vi "FormatLog.vi"(6 "log input":string, 8 "error in (no error)":errorcluster, 9 "System":string, 10 "Type":T1(ring), 11 "Log in":refnum<class "Log.lvclass">) -> (0 "error out":errorcluster, 3 "Log out":refnum<class "Log.lvclass">)   [LabVIEW 2018, in "Log.lvclass"]
uses:
  Log.lvclass
  Log.lvclass/Log.ctl
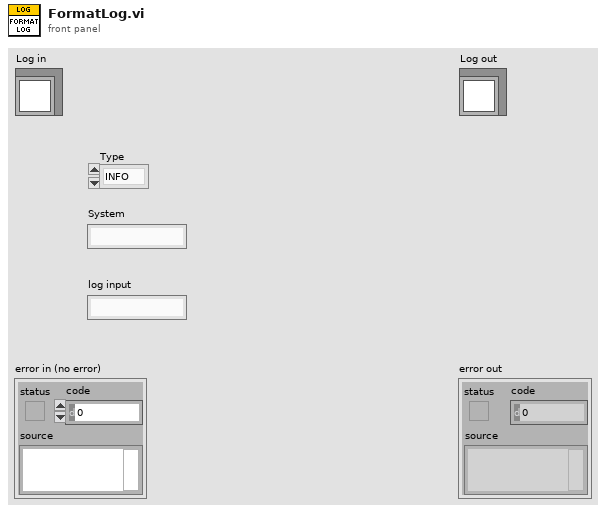
[diagram p1: front panel]
types:
  T1 = enum16{"INFO ", "TRACE", "DEBUG", "WARN ", "ERROR", "FATAL", "OTHER"}
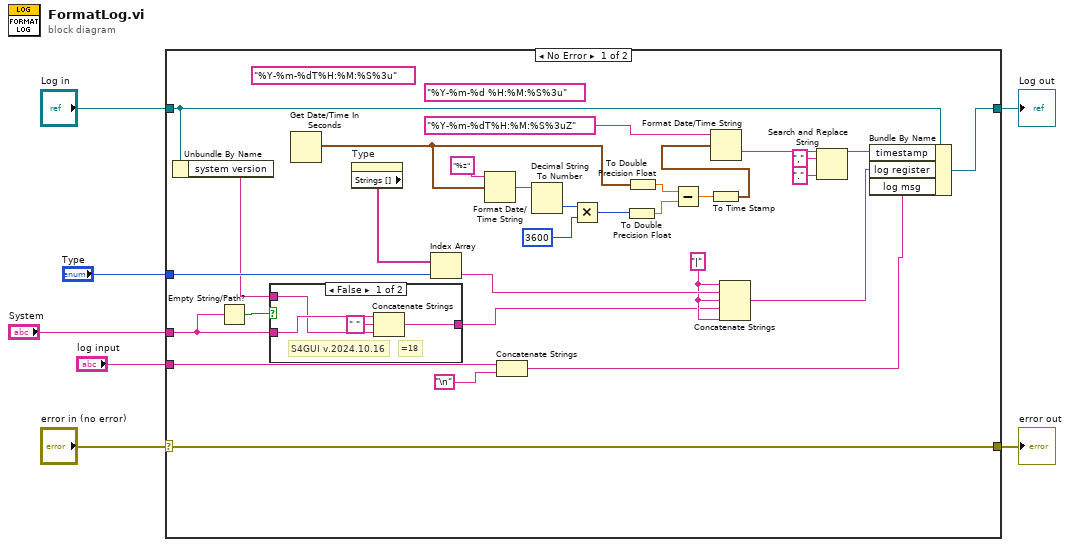
[diagram p0: block diagram]
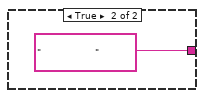
[diagram p2: hidden frame]
diagram:
  n1 = case shown="No Error" "error in (no error)" {
    selector: "error in (no error)" -> [w37 w44]
    tunnel: [w37 w44] -> w6
    tunnel: [w31 w43] -> w5
    tunnel: "Log in" -> [w23 w43]
    tunnel: "Type" -> [w35 _]
    tunnel: "log input" -> [w26 _]
    tunnel: "System" -> [w19 _]
    frame No Error {
      (unwired) "%Y-%m-%d %H:%M:%S%3u" ("time format string (%c)")
      w28 = "|" ("string")
      (unwired) "%Y-%m-%dT%H:%M:%S%3u" ("time format string (%c)")
      n2 = Unbundle By Name(w23) -> ("system version"=w20:string)
      n3 = Empty String/Path?(string/path=w19) -> (empty?=w22:bool)
      n4 = case shown="False" w22 {
        tunnel: [w38 "                  " ("t")] -> w21
        tunnel: w20 -> [w39 _]
        tunnel: w19 -> [w41 _]
        frame False {
          # "=18"
          # "S4GUI v.2024.10.16"
          n5 = Concatenate Strings(w41, " " ("string"), w39) -> (w38:string)
        }
        frame True {
        }
      }
      n6 = Get Date/Time In Seconds() -> (seconds since 1Jan1904=w9:timestamp)
      n7 = property on="Type" class="Enum (strict)"() -> ("Strings []"=w36:string[])  [unwired: 2 in, 2 out]
      n8 = Index Array(array=w36, index=w35) -> (element=w29:string)
      n9 = Format Date/Time String(time format string (%c)="%z", seconds (now)=w9) -> (date/time string=w16:string)  [unwired: 1 in]
      n10 = Concatenate Strings(w26, "\n" ("string")) -> (w24:string)
      n11 = Decimal String To Number(string=w16) -> (number=w15:i32)  [unwired: 2 in, 1 out]
      n12 = Multiply(x=w15, y=3600) -> (x*y=w13:i32)
      n13 = To Double Precision Float(number=w13) -> (double precision float=w11:dbl)
      n14 = To Double Precision Float(number=w9) -> (double precision float=w12:dbl)
      n15 = Subtract(x=w12, y=w11) -> (x-y=w10:dbl)
      n16 = To Time Stamp(1:w10) -> (0:w8:timestamp)
      n17 = Format Date/Time String(time format string (%c)="%Y-%m-%dT%H:%M:%S%3uZ", seconds (now)=w8) -> (date/time string=w34:string)  [unwired: 1 in]
      n18 = Concatenate Strings(w28, w29, w28, w21, w28) -> (w27:string)
      n19 = Search and Replace String(input string=w34, search string=",", replace string="." ("replace string (\"\")")) -> (result string=w30:string)  [unwired: 5 in, 3 out]
      n20 = Bundle By Name(cluster=w23, "timestamp"=w30, "log register"=w27, "log msg"=w24) -> (w31:refnum<class "Log.lvclass">)
    }
    frame Error {
    }
  }
  "error out" <- w6
  "Log out" <- w5
